vi "rmFileIfExist.vi"(8 "error in (no error)":errorcluster, 11 "path":path) -> (0 "error out":errorcluster, 3 "pathDup":path)   [LabVIEW 2018]
doc: "Remove the file if it exists."
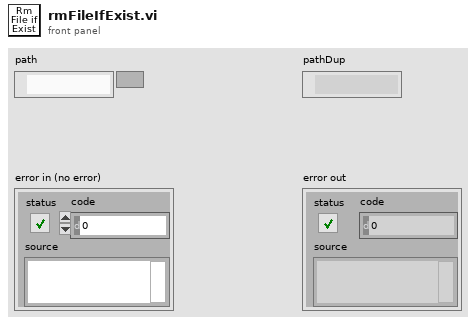
[diagram p1: front panel]
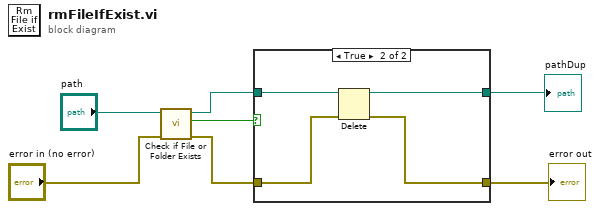
[diagram p0: block diagram]
diagram:
  n1 = call <vilib>:"Check if File or Folder Exists.vi"("error in (no error)"="error in (no error)", "path"="path") -> ("error out"=w3:errorcluster, "file or folder exists?"=w5:bool, "dup path"=w4:path)  [unwired: 7 in]
  n2 = case shown="True" w5 {
    tunnel: w4 -> [w9 w13]
    tunnel: w3 -> [w8 w12]
    tunnel: [w8 w11] -> w1
    tunnel: [w9 w10] -> w2
    frame False {
    }
    frame True {
      n3 = Delete(path (use dialog)=w13, error in=w12) -> (deleted path=w10:path, error out=w11:errorcluster)  [unwired: 3 in, 1 out]
    }
  }
  "error out" <- w1
  "pathDup" <- w2
